vi "createRatio.vi"(8 "error in (no error)":errorcluster, 9 "Denominator":i32, 10 "Numerator":i32, 11 "IRatio in":refnum<class "IRatio.lvclass">) -> (0 "error out":errorcluster, 3 "IRatio out":refnum<class "IRatio.lvclass">)   [LabVIEW 2022 SP3, in "openDAQ.lvlib" / "daqCoreTypes.lvlib" / "IRatio.lvclass"]
uses:
  <instrlib>/openDAQ/Public/Classes/daqCoreTypes/IRatio/IRatio.lvclass
  C:/Program Files (x86)/National Instruments/LabVIEW 2022/instr.lib/openDAQ/Public/Classes/IBaseObject/IBaseObject.lvclass
  <instrlib>/openDAQ/Public/Classes/IBaseObject/IBaseObject.lvclass/IBaseObject.ctl
  <instrlib>/openDAQ/Public/Classes/IBaseObject/Accessor/Read reference.vi
  <instrlib>/openDAQ/Public/Classes/IBaseObject/Accessor/Write reference.vi
  <instrlib>/openDAQ/Binaries/Windows/x86/copendaq32.dll
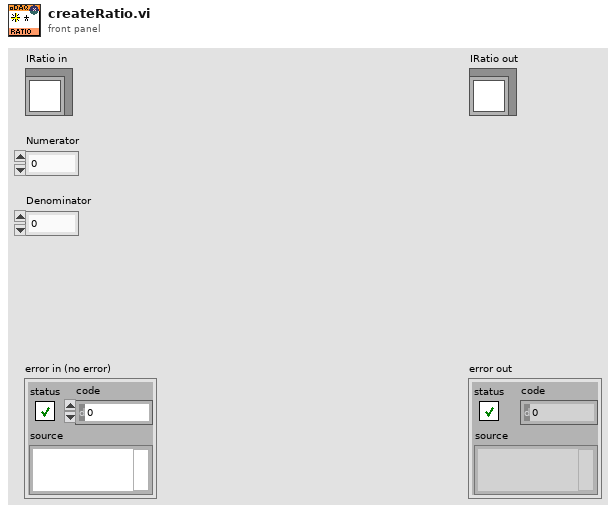
[diagram p1: front panel]
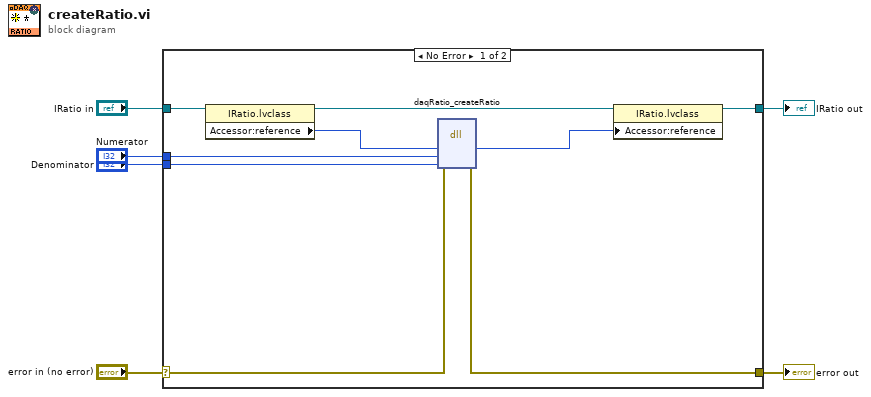
[diagram p0: block diagram]
diagram:
  n1 = case shown="No Error" "error in (no error)" {
    selector: "error in (no error)" -> [w15 w17]
    tunnel: [w14 w17] -> w5
    tunnel: [w10 w16] -> w3
    tunnel: "IRatio in" -> [w13 w16]
    tunnel: "Numerator" -> [w8 _]
    tunnel: "Denominator" -> [w7 _]
    frame No Error {
      n2 = property class="IRatio.lvclass"(reference=w13) -> (reference out=w11:refnum<class "IRatio.lvclass">, "Accessor:reference"=w12:i64)  [unwired: 1 in, 1 out]
      n3 = dll-call lib="C:/Program Files (x86)/National Instruments/LabVIEW 2022/instr.lib/openDAQ/Binaries/Windows/x86/copendaq*.*" fn="daqRatio_createRatio"(error in=w15, "daqString"=w12, "numerator"=w8, "denominator"=w7) -> (error out=w14:errorcluster, "daqString"=w9:i64)  [unwired: 5 in, 1 out]
      n4 = property class="IRatio.lvclass"(reference=w11, "Accessor:reference"=w9) -> (reference out=w10:refnum<class "IRatio.lvclass">)  [unwired: 1 in, 1 out]
    }
    frame Error {
    }
  }
  "error out" <- w5
  "IRatio out" <- w3
